vi "Write Value.vi"(8 "error in (no error)":errorcluster, 10 "Value":bool, 11 "int32 in":refnum<class "bool.lvclass">) -> (0 "error out":errorcluster, 3 "int32 out":refnum<class "bool.lvclass">)   [LabVIEW 2020, in "Protobuf RAW.lvlib" / "bool.lvclass"]
uses:
  bool.lvclass
  bool.lvclass/bool.ctl
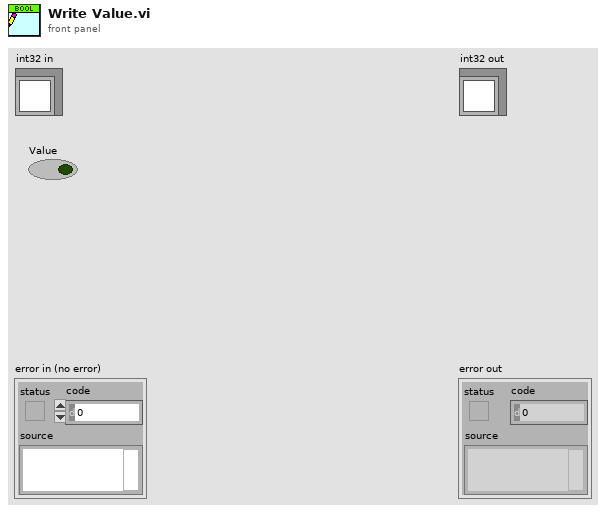
[diagram p1: front panel]
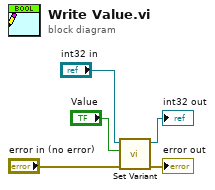
[diagram p0: block diagram]
diagram:
  n1 = call-dynamic "Set Variant.vi"("error in (no error)"="error in (no error)", "Variant"="Value", "int32 in"="int32 in") -> ("error out"=→"error out":errorcluster, "int32 out"=→"int32 out":refnum<class "bool.lvclass">)  [unwired: 7 in]
